vi "Read States.vi"(8 "error in (no error)":errorcluster, 11 "DefendGoalTacticVSS in":refnum<class "DefendGoalTacticVSS.lvclass">) -> (0 "error out":errorcluster, 2 "States":T1=enum."DefBallPos", 3 "DefendGoalTacticVSS out":refnum<class "DefendGoalTacticVSS.lvclass">)   [LabVIEW 2023, in "DefendGoalTacticVSS.lvclass"]
uses:
  DefendGoalTacticVSS.lvclass
  DefendGoalStates.ctl
  DefendGoalTacticVSS.lvclass/DefendGoalTacticVSS.ctl
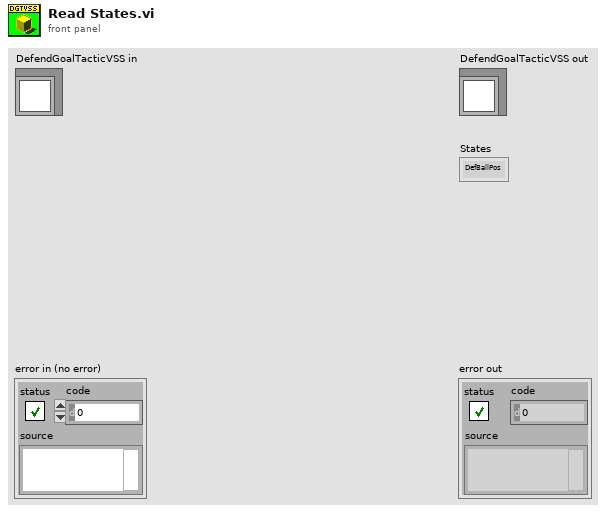
[diagram p1: front panel]
types:
  T1 = typedef "DefendGoalStates.ctl" = enum16{"Kick", "DefBallPos", "SpillSkin", "Exit"}
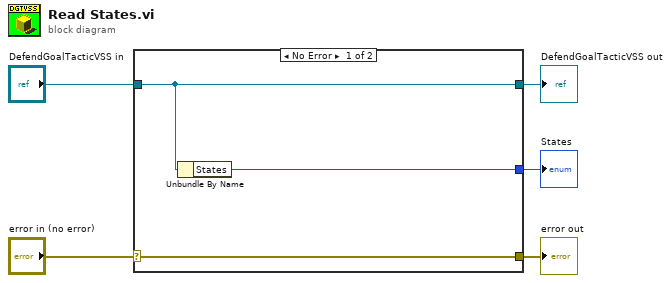
[diagram p0: block diagram]
diagram:
  n1 = case shown="No Error" "error in (no error)" {
    selector: "error in (no error)" -> [w8 w9]
    tunnel: [w8 w9] -> w4
    tunnel: [w7 w10] -> w2
    tunnel: "DefendGoalTacticVSS in" -> [w7 w10]
    tunnel: [w6 _] -> w1
    frame No Error {
      n2 = Unbundle By Name(w7) -> ("States"=w6:T1)
    }
    frame Error {
    }
  }
  "error out" <- w4
  "DefendGoalTacticVSS out" <- w2
  "States" <- w1
